vi "Predict GB Dimensions.vi"(9 "Mutual Viewing Angle":dbl[](array[numeric])=[1.0, 0.0, 0.0], 10 "Tolerance":dbl=0.001, 11 "Grain Boundary Macro Definition":T3={"Grain 1 Orientation"=[1.0, 0.6019417241891012, 0.029651947654046266], "Grain 2 Orientation"=[1.0, 0.730727623275494, 0.2205637301176], "Twist Angle (Deg)"=0.0}) -> (1 "Height Error":dbl, 2 "Width Error":dbl, 3 "Suggested Dimensions":T1)   [LabVIEW 2010]
uses:
  <vilib>/Analysis/Matrix/Datatypes/RealMatrix.ctl
  <vilib>/Analysis/baseanly.llb/Real A x B.vi
  <vilib>/Analysis/baseanly.llb/A x Vector.vi
  <vilib>/Analysis/NI_AALPro.lvlib
  <vilib>/Analysis/NI_AALBase.lvlib
  <vilib>/Analysis/Matrix/NI_Matrix.lvlib
panel:
  out "System Numeric Array":dbl[][](array[numeric])
  out "Suggested Dimensions 2":T1
  out "Grain 2 Height":dbl
  out "Grain 1 Height":dbl
  out "Grain 2 Width":dbl
  out "Grain 1 Width":dbl
  in  "Lattice Parameter":dbl=6.615785553057252
  out "Try this height":dbl
  out "Try this width":dbl
  out "Suggested X 2":dbl
  out "Suggested Y 2":dbl
  out "Suggested Grain 2 Length":dbl
  out "Suggested Grain 1 Length":dbl
  out "Suggested Y":dbl
  out "Suggested X":dbl
  out "Grain A":T2
  out "Grain B":T2
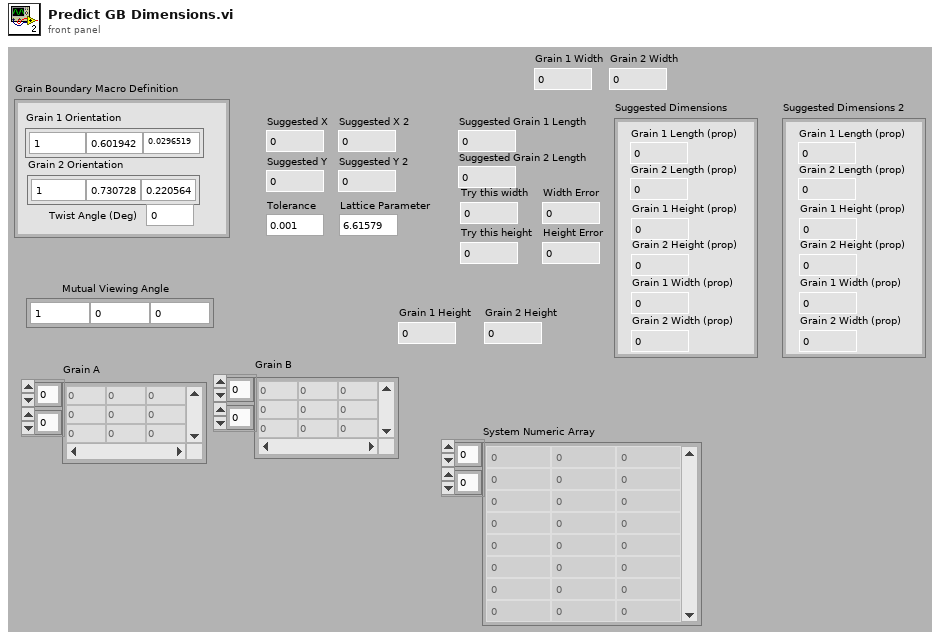
[diagram p1: front panel]
types:
  T1 = cluster{"Grain 1 Length (prop)":dbl, "Grain 2 Length (prop)":dbl, "Grain 1 Height (prop)":dbl, "Grain 2 Height (prop)":dbl, "Grain 1 Width (prop)":dbl, "Grain 2 Width (prop)":dbl}
  T2 = typedef "NI_Matrix.lvlib/RealMatrix.ctl" = dbl[][]
  T3 = cluster{"Grain 1 Orientation":dbl[], "Grain 2 Orientation":dbl[], "Twist Angle (Deg)":dbl}
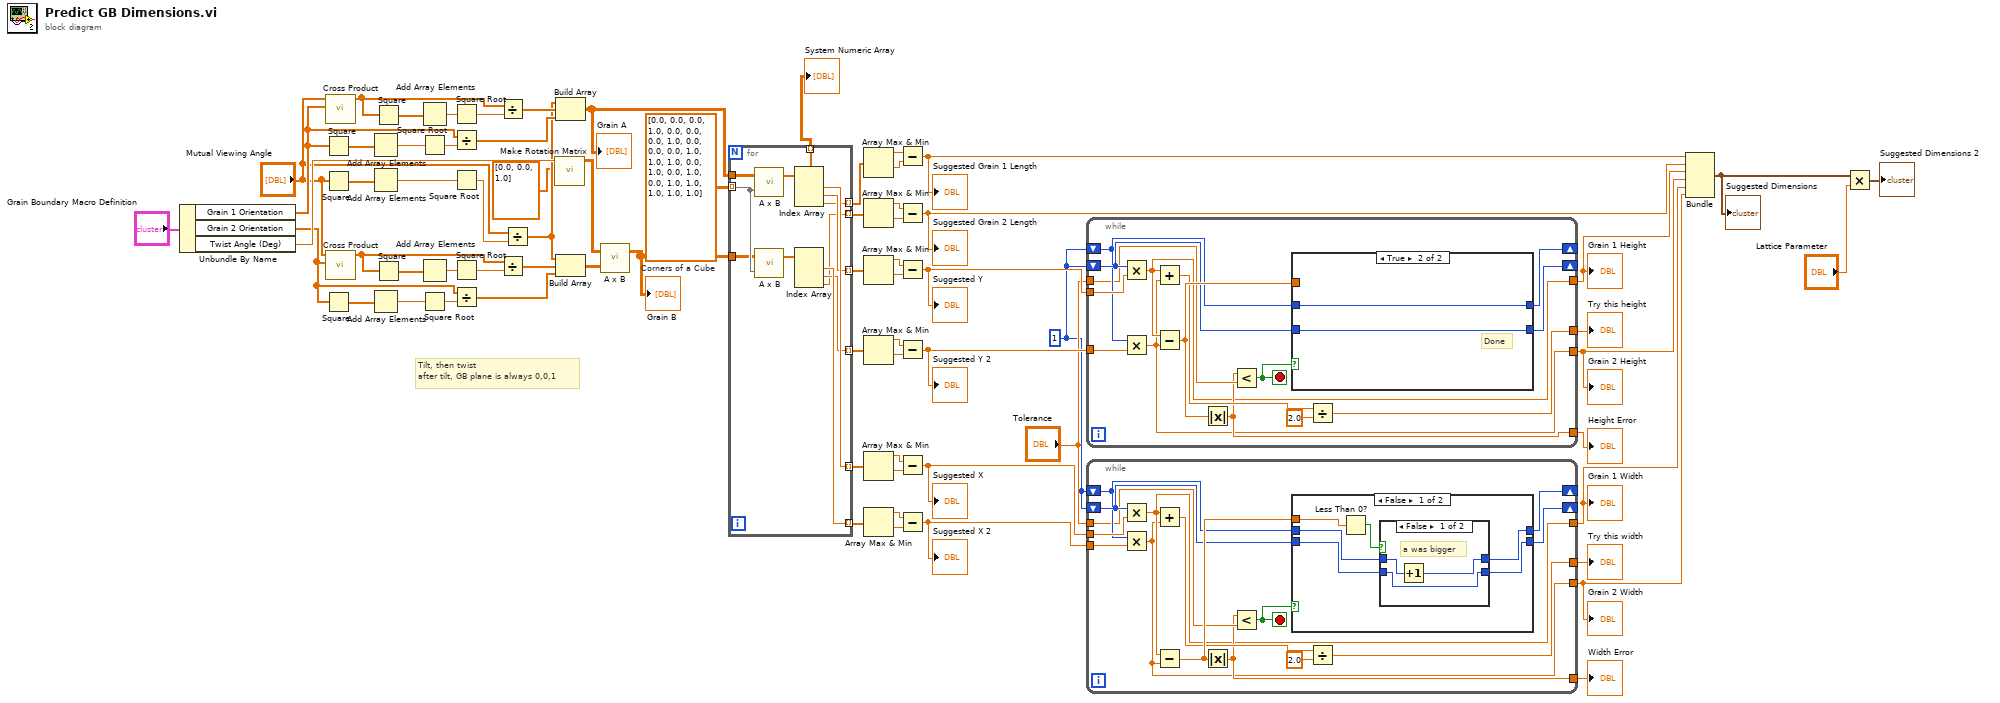
[diagram p0: block diagram]
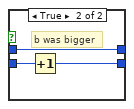
[diagram p2: hidden frame]
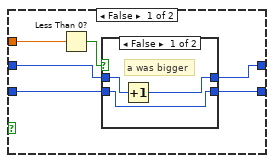
[diagram p4: hidden frame]
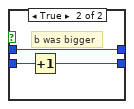
[diagram p5: hidden frame]
diagram:
  w63 = dbl[][] [[0.0, 0.0, 0.0], [1.0, 0.0, 0.0], [0.0, 1.0, 0.0], [0.0, 0.0, 1.0], [1.0, 1.0, 0.0], [1.0, 0.0, 1.0], [0.0, 1.0, 1.0], [1.0, 1.0, 1.0]]  # Corners of a Cube
  w37 = 1
  # "Tilt, then twist\nafter tilt, GB plane is always 0,0,1"
  n1 = Unbundle By Name("Grain Boundary Macro Definition") -> ("Grain 1 Orientation"=w23:dbl[], "Grain 2 Orientation"=w3:dbl[], "Twist Angle (Deg)"=w65:dbl)
  n2 = Square(x=w23) -> (x^2=w22:dbl[])
  n3 = Square(x="Mutual Viewing Angle") -> (x^2=w18:dbl[])
  n4 = Square(x=w3) -> (x^2=w4:dbl[])
  n5 = call <vilib>:"Cross Product.vi"("B Vector"=w23, "A Vector"="Mutual Viewing Angle") -> ("Cross Product"=w12:dbl[])  [unwired: 8 in, 1 out]
  n6 = call <vilib>:"Cross Product.vi"("B Vector"=w3, "A Vector"="Mutual Viewing Angle") -> ("Cross Product"=w8:dbl[])  [unwired: 8 in, 1 out]
  n7 = Add Array Elements(numeric array=w22) -> (sum=w21:dbl)
  n8 = Add Array Elements(numeric array=w18) -> (sum=w19:dbl)
  n9 = Add Array Elements(numeric array=w4) -> (sum=w5:dbl)
  n10 = Square(x=w12) -> (x^2=w14:dbl[])
  n11 = Square(x=w8) -> (x^2=w10:dbl[])
  n12 = Add Array Elements(numeric array=w14) -> (sum=w13:dbl)
  n13 = Square Root(x=w21) -> (sqrt(x)=w20:dbl)
  n14 = Add Array Elements(numeric array=w10) -> (sum=w9:dbl)
  n15 = Square Root(x=w5) -> (sqrt(x)=w2:dbl)
  n16 = Square Root(x=w13) -> (sqrt(x)=w11:dbl)
  n17 = Divide(x=w23, y=w20) -> (x/y=w71:dbl[])
  n18 = Square Root(x=w19) -> (sqrt(x)=w15:dbl)
  n19 = Square Root(x=w9) -> (sqrt(x)=w7:dbl)
  n20 = Divide(x=w3, y=w2) -> (x/y=w67:dbl[])
  n21 = Divide(x=w12, y=w11) -> (x/y=w70:dbl[])
  n22 = Divide(x=w8, y=w7) -> (x/y=w69:dbl[])
  n23 = Divide(x="Mutual Viewing Angle", y=w15) -> (x/y=w17:dbl[])
  n24 = call "Make Rotation Matrix.vi"("Rotation Axis"=dbl[] [0.0, 0.0, 1.0], "Rotation Angle (Degree)"=w65) -> ("Rotation Matrix"=w68:T2)  [unwired: 9 in]
  n25 = Build Array(w17, w70, w71) -> (w62:T2)
  "Grain A" <- w62
  n26 = Build Array(w17, w69, w67) -> (w66:T2)
  n27 = call-poly <vilib>:"A x B.vi"("B"=w66, "A"=w68) -> ("A x B"=w61:T2)  [unwired: 1 out]
  "Grain B" <- w61
  n28 = for {
    tunnel: w63 -> [w81] mode=indexing
    tunnel: w62 -> [w82]
    tunnel: w61 -> [w80]
    tunnel: [w78] -> w54 mode=indexing
    tunnel: [w77] -> w53 mode=indexing
    tunnel: [w76] -> w52 mode=indexing
    tunnel: [w75] -> w45 mode=indexing
    tunnel: [w74] -> w44 mode=indexing
    tunnel: [w73] -> w43 mode=indexing
    tunnel: [w72] -> w1 mode=indexing
    n29 = call-poly <vilib>:"A x B.vi"("Vector"=w81, "A"=w82) -> ("A x Vector"=w72:dbl[])  [unwired: 1 out]
    n30 = call-poly <vilib>:"A x B.vi"("Vector"=w81, "A"=w80) -> ("A x Vector"=w79:dbl[])  [unwired: 1 out]
    n31 = Index Array(array=w72) -> (element #1=w78:dbl, element #2=w77:dbl, element #3=w76:dbl)  [unwired: 3 in]
    n32 = Index Array(array=w79) -> (element #1=w75:dbl, element #2=w74:dbl, element #3=w73:dbl)  [unwired: 3 in]
  }
  "System Numeric Array" <- w1
  n33 = Array Max & Min(array=w52) -> (max value=w56:dbl, min value=w55:dbl)  [unwired: 2 out]
  n34 = Array Max & Min(array=w43) -> (max value=w50:dbl, min value=w51:dbl)  [unwired: 2 out]
  n35 = Array Max & Min(array=w53) -> (max value=w57:dbl, min value=w58:dbl)  [unwired: 2 out]
  n36 = Array Max & Min(array=w44) -> (max value=w49:dbl, min value=w48:dbl)  [unwired: 2 out]
  n37 = Array Max & Min(array=w54) -> (max value=w60:dbl, min value=w59:dbl)  [unwired: 2 out]
  n38 = Array Max & Min(array=w45) -> (max value=w46:dbl, min value=w47:dbl)  [unwired: 2 out]
  n39 = Subtract(x=w56, y=w55) -> (x-y=w35:dbl)
  "Suggested Grain 1 Length" <- w35
  n40 = Subtract(x=w50, y=w51) -> (x-y=w34:dbl)
  "Suggested Grain 2 Length" <- w34
  n41 = Subtract(x=w57, y=w58) -> (x-y=w42:dbl)
  "Suggested Y" <- w42
  n42 = Subtract(x=w49, y=w48) -> (x-y=w41:dbl)
  "Suggested Y 2" <- w41
  n43 = Subtract(x=w60, y=w59) -> (x-y=w39:dbl)
  "Suggested X" <- w39
  n44 = Subtract(x=w46, y=w47) -> (x-y=w38:dbl)
  "Suggested X 2" <- w38
  n45 = while {
    shift-right: [w92] -> _
    shift-left: w37 -> [w93]
    shift-right: [w90] -> _
    shift-left: w37 -> [w91]
    tunnel: w42 -> [w97]
    tunnel: w41 -> [w96]
    tunnel: [w86] -> w33
    tunnel: "Tolerance" -> [w89]
    tunnel: [w85] -> w36
    tunnel: [w84] -> w29
    tunnel: [w83] -> w28
    stop <- w95 stop-if-true
    n46 = Multiply(x=w93, y=w97) -> (x*y=w84:dbl)
    n47 = Multiply(x=w91, y=w96) -> (x*y=w83:dbl)
    n48 = Add(x=w84, y=w83) -> (x+y=w87:dbl)
    n49 = Subtract(x=w84, y=w83) -> (x-y=w94:dbl)
    n50 = Absolute Value(x=w94) -> (abs(x)=w85:dbl)
    n51 = Less?(x=w85, y=w89) -> (x < y?=w95:bool)
    n52 = case shown="True" w95 {
      tunnel: w94 -> [w103 _]
      tunnel: w93 -> [w102 w111]
      tunnel: [w101 w111] -> w92
      tunnel: w91 -> [w100 w110]
      tunnel: [w99 w110] -> w90
      frame False {
        n53 = Less Than 0?(x=w103) -> (x < 0?=w98:bool)
        n54 = case shown="False" w98 {
          tunnel: w102 -> [w104 w109]
          tunnel: [w104 w108] -> w101
          tunnel: w100 -> [w106 w107]
          tunnel: [w105 w107] -> w99
          frame False {
            # "a was bigger"
            n55 = Increment(x=w106) -> (x+1=w105:i32)
          }
          frame True {
            # "b was bigger"
            n56 = Increment(x=w109) -> (x+1=w108:i32)
          }
        }
      }
      frame True {
        # "Done"
      }
    }
    n57 = Divide(x=w87, y=2.0) -> (x/y=w86:dbl)
  }
  "Try this height" <- w33
  "Height Error" <- w36
  "Grain 1 Height" <- w29
  "Grain 2 Height" <- w28
  n58 = while {
    shift-right: [w121] -> _
    shift-left: w37 -> [w122]
    shift-right: [w119] -> _
    shift-left: w37 -> [w120]
    tunnel: w39 -> [w126]
    tunnel: w38 -> [w125]
    tunnel: [w115] -> w31
    tunnel: "Tolerance" -> [w118]
    tunnel: [w114] -> w32
    tunnel: [w113] -> w27
    tunnel: [w112] -> w26
    stop <- w124 stop-if-true
    n59 = Multiply(x=w122, y=w126) -> (x*y=w113:dbl)
    n60 = Multiply(x=w120, y=w125) -> (x*y=w112:dbl)
    n61 = Add(x=w113, y=w112) -> (x+y=w116:dbl)
    n62 = Subtract(x=w113, y=w112) -> (x-y=w123:dbl)
    n63 = Absolute Value(x=w123) -> (abs(x)=w114:dbl)
    n64 = Less?(x=w114, y=w118) -> (x < y?=w124:bool)
    n65 = case shown="False" w124 {
      tunnel: w123 -> [w132 _]
      tunnel: w122 -> [w131 w140]
      tunnel: [w130 w140] -> w121
      tunnel: w120 -> [w129 w139]
      tunnel: [w128 w139] -> w119
      frame False {
        n66 = Less Than 0?(x=w132) -> (x < 0?=w127:bool)
        n67 = case shown="False" w127 {
          tunnel: w131 -> [w133 w138]
          tunnel: [w133 w137] -> w130
          tunnel: w129 -> [w135 w136]
          tunnel: [w134 w136] -> w128
          frame False {
            # "a was bigger"
            n68 = Increment(x=w135) -> (x+1=w134:i32)
          }
          frame True {
            # "b was bigger"
            n69 = Increment(x=w138) -> (x+1=w137:i32)
          }
        }
      }
      frame True {
        # "Done"
      }
    }
    n70 = Divide(x=w116, y=2.0) -> (x/y=w115:dbl)
  }
  "Try this width" <- w31
  "Width Error" <- w32
  "Grain 1 Width" <- w27
  "Grain 2 Width" <- w26
  n71 = Bundle(w35, w34, w29, w28, w27, w26) -> (w25:cluster{dbl, dbl, dbl, dbl, dbl, dbl})  [unwired: 1 in]
  "Suggested Dimensions" <- w25
  n72 = Multiply(x=w25, y="Lattice Parameter") -> (x*y=→"Suggested Dimensions 2":cluster{dbl, dbl, dbl, dbl, dbl, dbl})
